vi "HH_ToImage.vi"(0 "Data In":u32[](array[numeric]), 1 "Reset":bool, 2 "Image Array In":i32[][](array[numeric]), 5 "Data Count":i32, 9 "Pixel Time (Laser Pulses)":i32=25, 11 "Trace Bins":i32=25) -> (3 "Image Array Out":i32[][](array[numeric]), 4 "Histograms":i32[][](array[numeric]), 6 "Total Photon Count":u64[](array[numeric]), 8 "Trigger Times":u64[](array[numeric]), 13 "Total Oveflow Count":u64, 14 "Num Records Total":i64, 15 "Traces":i32[][](array[numeric]))   [LabVIEW 2013]
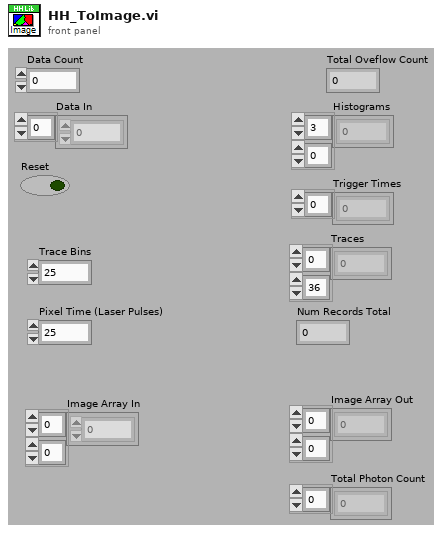
[diagram p1: front panel]
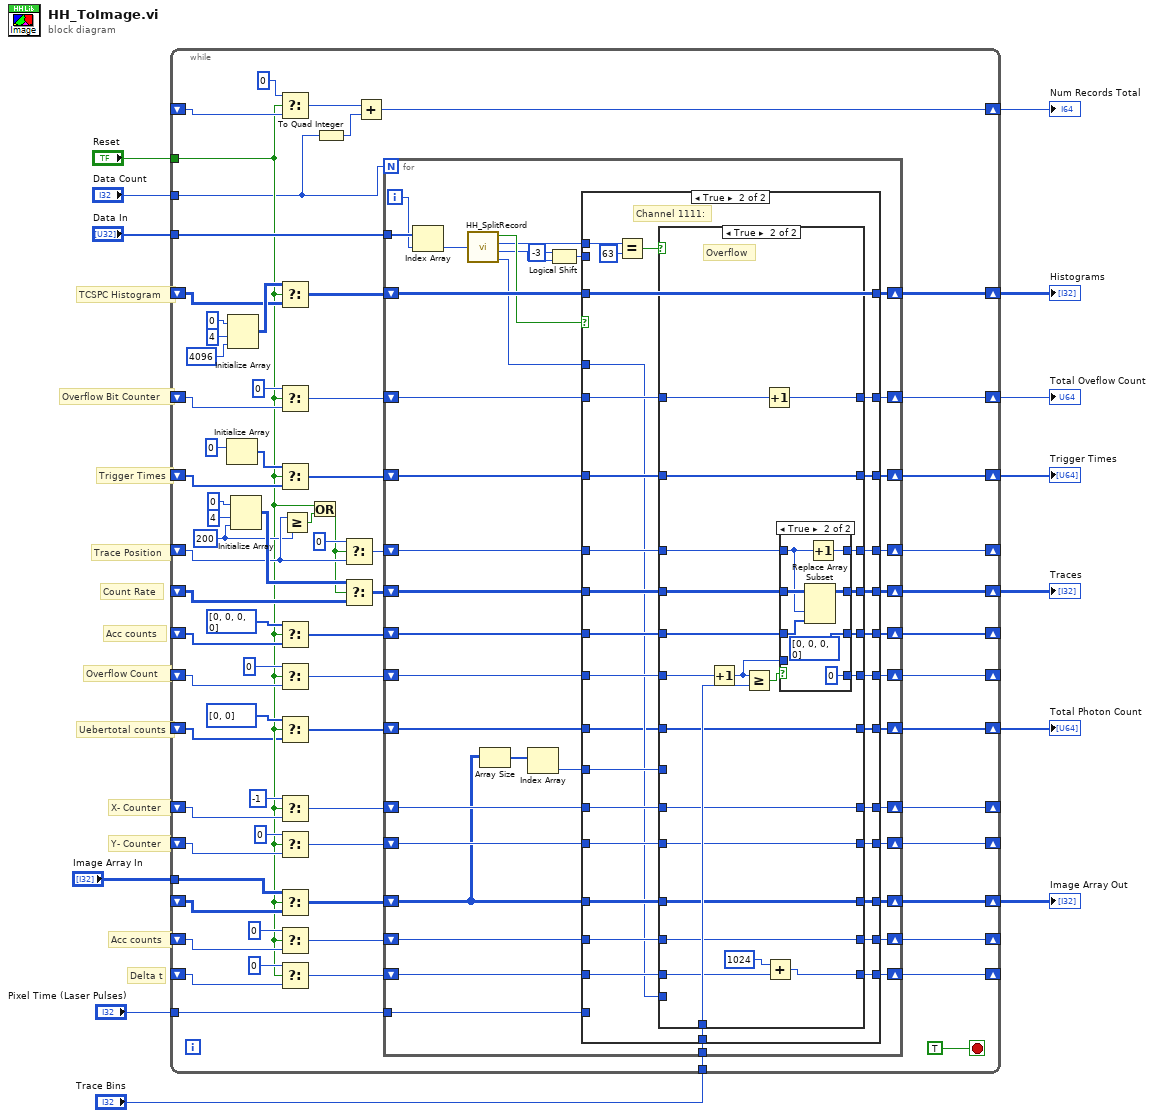
[diagram p0: block diagram]
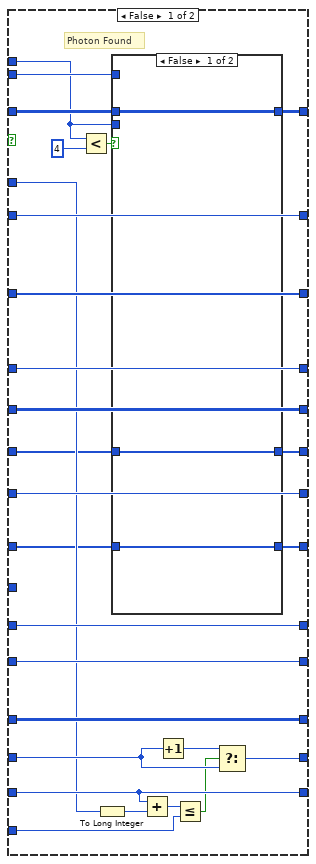
[diagram p2: hidden frame]
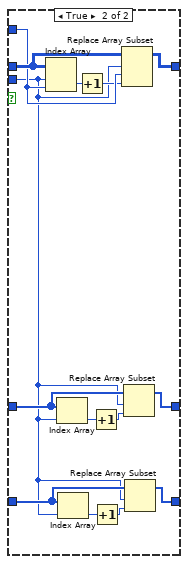
[diagram p3: hidden frame]
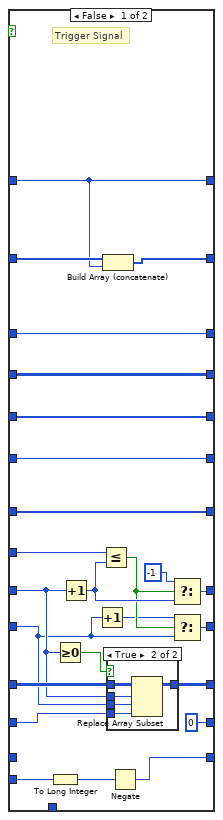
[diagram p4: hidden frame]
diagram:
  # "Uebertotal counts"
  # "Y- Counter"
  # "X- Counter"
  # "Delta t"
  # "Acc counts"
  # "Trace Position"
  # "Overflow Count"
  # "Acc counts"
  # "Count Rate"
  # "Trigger Times"
  # "TCSPC Histogram"
  # "Overflow Bit Counter"
  n1 = while {
    tunnel: "Data In" -> [w83]
    shift-right: [w84] -> w13
    shift-left: _ -> [w79]
    tunnel: "Reset" -> [w19]
    shift-right: [w76] -> w2
    shift-left: _ -> [w75]
    shift-right: [w71] -> w10
    shift-left: _ -> [w70]
    shift-right: [w66] -> w8
    shift-left: _ -> [w65]
    shift-right: [w63] -> _
    shift-left: _ -> [w62]
    shift-right: [w60] -> _
    shift-left: _ -> [w59]
    tunnel: "Trace Bins" -> [w58]
    shift-right: [w55] -> _
    shift-left: _ -> [w53]
    shift-right: [w49] -> w5
    shift-left: _ -> [w48]
    tunnel: "Image Array In" -> [w51]
    shift-right: [w44] -> _
    shift-left: _ -> [w42]
    shift-right: [w43] -> _
    shift-left: _ -> [w41]
    tunnel: "Pixel Time (Laser Pulses)" -> [w40]
    shift-right: [w35] -> _
    shift-left: _ -> [w33]
    shift-right: [w34] -> _
    shift-left: _ -> [w32]
    tunnel: "Data Count" -> [w15]
    shift-right: [w27] -> w3
    shift-left: _ -> [w29]
    shift-right: [w17] -> w1
    shift-left: _ -> [w16]
    stop <- TRUE stop-if-true
    w24 = 200 ("dimension size")
    n2 = Initialize Array(u64 0 ("element")) -> (w73:u64[])  [unwired: 1 in]
    n3 = Initialize Array(0 ("element"), 4 ("dimension size"), 4096 ("dimension size")) -> (w80:i32[][])
    n4 = Initialize Array(0 ("element"), 4 ("dimension size"), w24) -> (w68:i32[][])
    n5 = Select(t=i64 0 ("Data Count 2"), s=w19, f=w29) -> (s? t:f=w28:i64)
    n6 = Select(t=w80, s=w19, f=w79) -> (s? t:f=w81:i32[][])
    n7 = Select(t=u64 0, s=w19, f=w75) -> (s? t:f=w77:u64)
    n8 = Select(t=w73, s=w19, f=w70) -> (s? t:f=w72:u64[])
    n9 = Select(t=u32[] [0, 0, 0, 0] ("initialized array"), s=w19, f=w62) -> (s? t:f=w64:u32[])
    n10 = Select(t=u32 0, s=w19, f=w59) -> (s? t:f=w61:u32)
    n11 = Select(t=u64[] [0, 0] ("initialized array"), s=w19, f=w16) -> (s? t:f=w18:u64[])
    n12 = Select(t=-1, s=w19, f=w33) -> (s? t:f=w37:i32)
    n13 = Select(t=0, s=w19, f=w32) -> (s? t:f=w36:i32)
    n14 = Select(t=w51, s=w19, f=w48) -> (s? t:f=w50:i32[][])
    n15 = Select(t=0, s=w19, f=w42) -> (s? t:f=w46:i32)
    n16 = Select(t=0, s=w19, f=w41) -> (s? t:f=w45:i32)
    n17 = Greater Or Equal?(x=w53, y=w24) -> (x >= y?=w54:bool)
    n18 = Or(x=w19, y=w54) -> (x .or. y?=w52:bool)
    n19 = To Quad Integer(1:w15) -> (0:w14:i64)
    n20 = Select(t=0, s=w52, f=w53) -> (s? t:f=w56:i32)
    n21 = Select(t=w68, s=w52, f=w65) -> (s? t:f=w67:i32[][])
    n22 = Add(x=w28, y=w14) -> (x+y=w27:i64)
    n23 = for {
      N: w15 -> [_]
      tunnel: w83 -> [w96]
      shift-right: [w123] -> w84
      shift-left: w81 -> [w124]
      shift-right: [w121] -> w76
      shift-left: w77 -> [w122]
      shift-right: [w119] -> w71
      shift-left: w72 -> [w120]
      shift-right: [w115] -> w66
      shift-left: w67 -> [w116]
      shift-right: [w117] -> w63
      shift-left: w64 -> [w118]
      shift-right: [w113] -> w60
      shift-left: w61 -> [w114]
      tunnel: w58 -> [w112]
      shift-right: [w110] -> w55
      shift-left: w56 -> [w111]
      shift-right: [w109] -> w49
      shift-left: w50 -> [w101]
      shift-right: [w107] -> w44
      shift-left: w46 -> [w108]
      shift-right: [w105] -> w43
      shift-left: w45 -> [w106]
      tunnel: w40 -> [w97]
      shift-right: [w102] -> w35
      shift-left: w37 -> [w103]
      shift-right: [w98] -> w34
      shift-left: w36 -> [w104]
      shift-right: [w93] -> w17
      shift-left: w18 -> [w94]
      i -> [w95]
      n24 = Index Array(array=w96, index=w95) -> (element=w92:u32)
      n25 = call "HH_SplitRecord.vi"("Record in"=w92) -> ("Special"=w91:bool, "channel"=w87:i32, "time"=w89:i32, "nsync"=w86:u16)
      n26 = Array Size(array=w101) -> (size(s)=w100:i32[])
      n27 = Index Array(array=w100) -> (element=w99:i32)  [unwired: 1 in]
      n28 = Logical Shift(y=i8 -3, x=w89) -> (x << y=w88:i32)
      n29 = case shown="True" w91 {
        tunnel: w124 -> [w151 w197]
        tunnel: w87 -> [w125 w170]
        tunnel: [w150 w197] -> w123
        tunnel: w88 -> [w126 _]
        tunnel: w122 -> [w149 w199]
        tunnel: [w149 w198] -> w121
        tunnel: w120 -> [w148 w196]
        tunnel: [w148 w195] -> w119
        tunnel: w118 -> [w132 w193]
        tunnel: [w131 w189] -> w117
        tunnel: w116 -> [w147 w192]
        tunnel: [w147 w188] -> w115
        tunnel: w114 -> [w146 w194]
        tunnel: [w146 w190] -> w113
        tunnel: w112 -> [_ w191]
        tunnel: w111 -> [w145 w187]
        tunnel: [w145 w186] -> w110
        tunnel: w101 -> [w144 w184]
        tunnel: [w144 w185] -> w109
        tunnel: w108 -> [w143 w180]
        tunnel: [w142 w181] -> w107
        tunnel: w106 -> [w141 w183]
        tunnel: [w141 w182] -> w105
        tunnel: w104 -> [w140 w179]
        tunnel: w103 -> [w139 w178]
        tunnel: [w139 w177] -> w102
        tunnel: w99 -> [_ w176]
        tunnel: [w140 w175] -> w98
        tunnel: w97 -> [w138 _]
        tunnel: w86 -> [w134 w174]
        tunnel: w94 -> [w128 w173]
        tunnel: [w127 w172] -> w93
        frame False {
          # "Photon Found"
          n30 = Less?(x=w125, y=4) -> (x < y?=w130:bool)
          n31 = To Long Integer(number=w134) -> (32bit integer=w133:i32)
          n32 = case shown="False" w130 {
            tunnel: w151 -> [w154 w168]
            tunnel: [w154 w167] -> w150
            tunnel: w126 -> [_ w166]
            tunnel: w125 -> [_ w155]
            tunnel: w132 -> [w153 w165]
            tunnel: [w153 w164] -> w131
            tunnel: w128 -> [w152 w157]
            tunnel: [w152 w156] -> w127
            frame False {
            }
            frame True {
              n33 = Index Array(array=w168, index (row)=w155, index (col)=w166) -> (element=w163:i32)
              n34 = Index Array(array=w165, index=w155) -> (element=w161:u32)
              n35 = Index Array(array=w157, index=w155) -> (element=w159:u64)
              n36 = Increment(x=w163) -> (x+1=w162:i32)
              n37 = Increment(x=w161) -> (x+1=w160:u32)
              n38 = Increment(x=w159) -> (x+1=w158:u64)
              n39 = Replace Array Subset(array=w168, new element=w162, index (row)=w155, index (col)=w166) -> (w167:i32[][])
              n40 = Replace Array Subset(array=w165, new element=w160, index=w155) -> (w164:u32[])
              n41 = Replace Array Subset(array=w157, new element=w158, index=w155) -> (w156:u64[])
            }
          }
          n42 = Add(x=w141, y=w133) -> (x+y=w135:i32)
          n43 = Increment(x=w143) -> (x+1=w137:i32)
          n44 = Less Or Equal?(x=w135, y=w138) -> (x <= y?=w136:bool)
          n45 = Select(t=w137, s=w136, f=w143) -> (s? t:f=w142:i32)
        }
        frame True {
          # "Channel 1111:"
          n46 = Equal?(x=w170, y=63) -> (x = y?=w169:bool)
          n47 = case shown="True" w169 {
            tunnel: w199 -> [w222 w251]
            tunnel: [w222 w250] -> w198
            tunnel: w196 -> [w224 w252]
            tunnel: [w223 w252] -> w195
            tunnel: w194 -> [w221 w235]
            tunnel: w193 -> [w220 w246]
            tunnel: w192 -> [w219 w244]
            tunnel: w191 -> [_ w249]
            tunnel: [w221 w247] -> w190
            tunnel: [w220 w245] -> w189
            tunnel: [w219 w243] -> w188
            tunnel: w187 -> [w218 w242]
            tunnel: [w218 w241] -> w186
            tunnel: [w215 w240] -> w185
            tunnel: w184 -> [w216 w240]
            tunnel: w183 -> [_ w233]
            tunnel: [w201 w231] -> w182
            tunnel: [0 ("t") w238] -> w181
            tunnel: w180 -> [w214 w238]
            tunnel: w174 -> [w217 _]
            tunnel: w179 -> [w204 w237]
            tunnel: w178 -> [w209 w236]
            tunnel: [w211 w236] -> w177
            tunnel: w176 -> [w210 _]
            tunnel: [w205 w237] -> w175
            tunnel: w173 -> [w200 w232]
            tunnel: [w200 w232] -> w172
            frame False {
              # "Trigger Signal"
              n48 = To Long Integer(number=w217) -> (32bit integer=w202:i32)
              n49 = Greater Or Equal To 0?(x=w209) -> (x >= 0?=w212:bool)
              n50 = Increment(x=w209) -> (x+1=w208:i32)
              n51 = Increment(x=w204) -> (x+1=w203:i32)
              n52 = Less Or Equal?(x=w210, y=w208) -> (x <= y?=w206:bool)
              n53 = Build Array (concatenate)(w224, w222) -> (w223:u64[])
              n54 = case shown="True" w212 {
                tunnel: w216 -> [w225 w230]
                tunnel: [w225 w229] -> w215
                tunnel: w214 -> [_ w228]
                tunnel: w204 -> [_ w227]
                tunnel: w209 -> [_ w226]
                frame False {
                }
                frame True {
                  n55 = Replace Array Subset(array=w230, new element=w228, index (row)=w226, index (col)=w227) -> (w229:i32[][])
                }
              }
              n56 = Negate(x=w202) -> (-x=w201:i32)
              n57 = Select(t=-1, s=w206, f=w208) -> (s? t:f=w211:i32)
              n58 = Select(t=w203, s=w206, f=w204) -> (s? t:f=w205:i32)
            }
            frame True {
              # "Overflow"
              n59 = Increment(x=w235) -> (x+1=w234:u32)
              n60 = Greater Or Equal?(x=w234, y=w249) -> (x >= y?=w248:bool)
              n61 = Increment(x=w251) -> (x+1=w250:u64)
              n62 = Add(x=1024 ("t"), y=w233) -> (x+y=w231:i32)
              n63 = case shown="True" w248 {
                tunnel: w234 -> [w256 _]
                tunnel: [w256 u32 0] -> w247
                tunnel: w246 -> [w255 w261]
                tunnel: [w255 u32[] [0, 0, 0, 0] ("initialized array")] -> w245
                tunnel: w244 -> [w254 w262]
                tunnel: [w254 w260] -> w243
                tunnel: w242 -> [w253 w258]
                tunnel: [w253 w259] -> w241
                frame False {
                }
                frame True {
                  n64 = Replace Array Subset(array=w262, new element=w261, index (col)=w258) -> (w260:i32[][])  [unwired: 1 in]
                  n65 = Increment(x=w258) -> (x+1=w259:i32)
                }
              }
            }
          }
        }
      }
    }
  }
  "Histograms" <- w13
  "Trigger Times" <- w10
  "Traces" <- w8
  "Image Array Out" <- w5
  "Num Records Total" <- w3
  "Total Oveflow Count" <- w2
  "Total Photon Count" <- w1
